vi "Write State.vi"(8 "error in (no error)":errorcluster, 10 "State":refnum<class "State Pattern.lvclass">, 11 "A State in":refnum<class "A State.lvclass">) -> (0 "error out":errorcluster, 3 "A State out":refnum<class "A State.lvclass">)   [LabVIEW 2021, in "Context.lvlib" / "A State.lvclass"]
uses:
  A State.lvclass
  State Pattern/State Pattern/State Pattern.lvclass
  Context/Context.lvclass
  A State.lvclass/A State.ctl
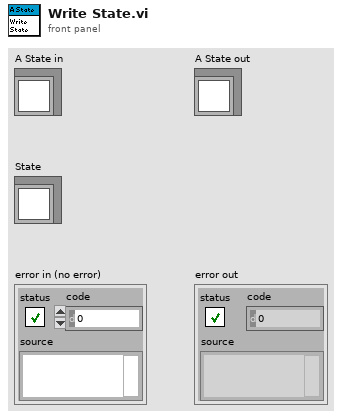
[diagram p1: front panel]
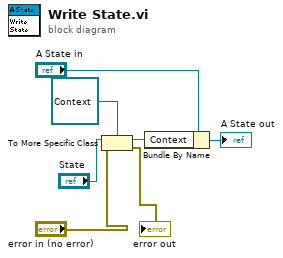
[diagram p0: block diagram]
diagram:
  n1 = To More Specific Class(target class=refnum<class "Context.lvclass"> refnum ("Context Actor.lvlib:Context Actor.lvclass"), reference="State", error in="error in (no error)") -> (specific class reference=w2:refnum<class "Context.lvclass">, error out=→"error out":errorcluster)
  n2 = Bundle By Name(cluster="A State in", "Context"=w2) -> (→"A State out":refnum<class "A State.lvclass">)
